vi "Right Subpanel_A.vi"() -> ()   [LabVIEW 2010]
panel:
  in  "Tree":string(tree)
  # "Right Subpanel_A.vi"
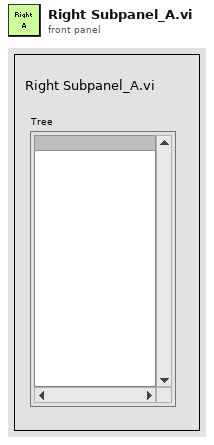
[diagram p1: front panel]
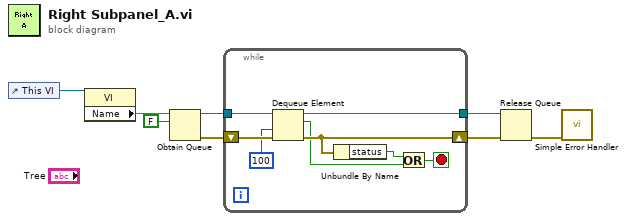
[diagram p0: block diagram]
diagram:
  n1 = control-ref of="This VI"() -> (w7:refnum<vi>)
  n2 = property class="VI"(reference=w7) -> ("Name"=w6:string)  [unwired: 1 in, 2 out]
  n3 = Obtain Queue(name (unnamed)=w6, element data type=FALSE) -> (queue out=w5:refnum<queue>, error out=w4:errorcluster)  [unwired: 3 in, 1 out]
  n4 = while {
    tunnel: w5 -> [w15]
    shift-right: [w12] -> w2
    shift-left: w4 -> [w16]
    tunnel: [w13] -> w3
    stop <- w10 stop-if-true
    n5 = Dequeue Element(queue=w15, timeout in ms (-1)=100, error in (no error)=w16) -> (queue out=w13:refnum<queue>, element=w11:bool, error out=w12:errorcluster)  [unwired: 1 out]
    n6 = Unbundle By Name(w12) -> ("status"=w9:bool)
    n7 = Or(x=w9, y=w11) -> (x .or. y?=w10:bool)
  }
  n8 = Release Queue(queue=w3, error in (no error)=w2) -> (error out=w1:errorcluster)  [unwired: 1 in, 2 out]
  n9 = call <vilib>:"Simple Error Handler.vi"("error in (no error)"=w1) -> ()  [unwired: 4 in, 5 out]
